vi "Multiply Polynomials (DBL).vi"(8 "threshold type":T1 items=["Absolute Value", "Relative Value"], 9 "threshold":dbl, 10 "Q(x)":dbl[](array[numeric]), 11 "P(x)":dbl[](array[numeric])) -> (0 "error":i32, 3 "P(x)*Q(x)":dbl[](array[numeric]))   [LabVIEW 2017, in "NI_AALPro.lvlib"]
doc: "Multiplies polynomial <B>P(x)</B> by polynomial <B>Q(x)</B>. The data types you wire to the <B>P(x)</B> and <B>Q(x)</B> inputs determine the polymorphic instance to use."
uses:
  <vilib>/Analysis/NI_AALPro.lvlib
  <vilib>/Analysis/polynomials.llb/Remove Zero Threshold Type.ctl
  <vilib>/Analysis/polynomials.llb/Remove Zero Coefficients (DBL).vi
  <resource>/lvanlys.dll
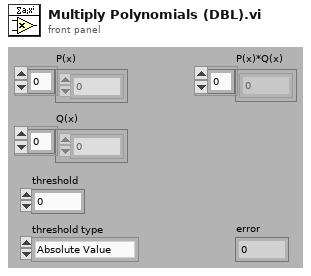
[diagram p1: front panel]
types:
  T1 = typedef "NI_AALPro.lvlib/Remove Zero Threshold Type.ctl" = u16
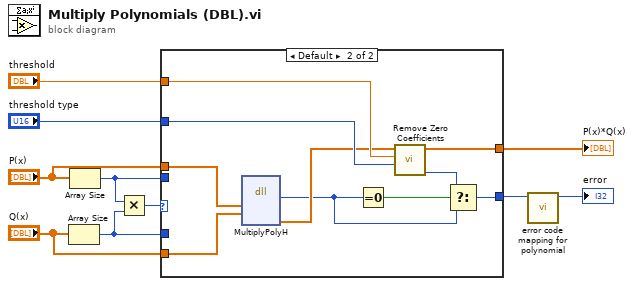
[diagram p0: block diagram]
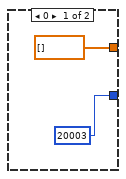
[diagram p2: hidden frame]
diagram:
  n1 = Array Size(array="Q(x)") -> (size(s)=w6:i32)
  n2 = Array Size(array="P(x)") -> (size(s)=w7:i32)
  n3 = Multiply(x=w7, y=w6) -> (x*y=w8:i32)
  n4 = case shown="Default" w8 {
    tunnel: w7 -> [_ _]
    tunnel: w6 -> [_ _]
    tunnel: "P(x)" -> [_ w16]
    tunnel: "Q(x)" -> [_ w15]
    tunnel: [dbl[] [] ("BDL") w20] -> w5
    tunnel: [20003 ("empty array") w21] -> w4
    tunnel: "threshold" -> [_ w18]
    tunnel: "threshold type" -> [_ w17]
    frame 0 {
    }
    frame Default {
      n5 = dll-call lib="e:/builds/penguin/labview/branches/2017/dev/dist/resource/lvanlys.*" fn="MultiplyPolyH"("pH"=w16, "qH"=w15) -> ("error"=w13:i32, "pqH"=w14:dbl[])  [unwired: 6 in, 2 out]
      n6 = Equal To 0?(x=w13) -> (x = 0?=w22:bool)
      n7 = call-poly <vilib>:"Remove Zero Coefficients.vi"("threshold type"=w17, "threshold"=w18, "P(x) In"=w14) -> ("error"=w19:i32, "P(x) Out"=w20:dbl[])  [unwired: 6 in, 1 out]
      n8 = Select(t=w19, s=w22, f=w13) -> (s? t:f=w21:i32)
    }
  }
  "P(x)*Q(x)" <- w5
  n9 = call <vilib>:"error code mapping for polynomial.vi"("error in"=w4) -> ("error out"=→"error":i32)  [unwired: 10 in]
